vi "switchtype.vi"() -> ()   [LabVIEW 2013]
panel:
  out "lvDataCluster.h":string
  in  "names":string[](array[string])=["Double", "Single", "I64", "I32", "I16", "I8", "U64", "U32", "U16", "U8", "Boolean", "String"]
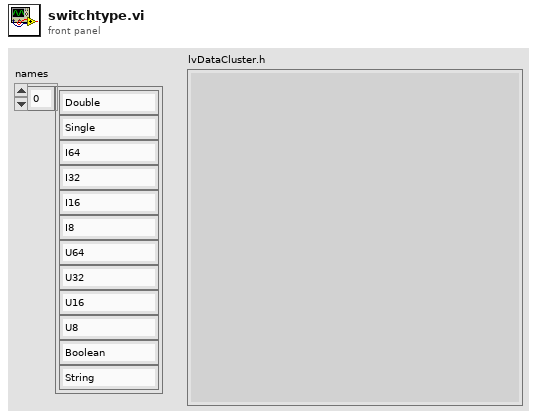
[diagram p1: front panel]
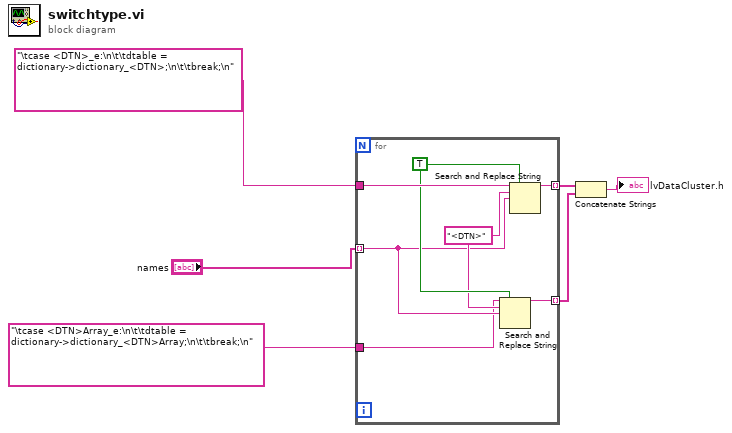
[diagram p0: block diagram]
diagram:
  n1 = for {
    tunnel: "names" -> [w9] mode=indexing
    tunnel: "\tcase <DTN>_e:\n\t\tdtable = dictionary->dictionary_<DTN>;\n\t\tbreak;\n" -> [w13]
    tunnel: [w12] -> w4 mode=indexing
    tunnel: [w8] -> w2 mode=indexing
    tunnel: "\tcase <DTN>Array_e:\n\t\tdtable = dictionary->dictionary_<DTN>Array;\n\t\tbreak;\n" -> [w7]
    w11 = TRUE ("replace all? (F)")
    w10 = "<DTN>"
    n2 = Search and Replace String(replace all?=w11, input string=w7, search string=w10, replace string=w9) -> (result string=w8:string)  [unwired: 4 in, 3 out]
    n3 = Search and Replace String(replace all?=w11, input string=w13, search string=w10, replace string=w9) -> (result string=w12:string)  [unwired: 4 in, 3 out]
  }
  n4 = Concatenate Strings(w4, w2) -> (→"lvDataCluster.h":string)
